vi "save_to_file.vi"(1 "Cell Settings Array 4":T1=[{"Measure?"=TRUE, "Area (cm^2)"=0.0, "Cell Label"="", "Cell Description"="", "Time between scans (s)"=0.0, "Cell Position"=1, "Scan settings in queue"=0, "Sample holder"=4.0, "User name"=""}, {"Measure?"=TRUE, "Area (cm^2)"=0.0, "Cell Label"="", "Cell Description"="", "Time between scans (s)"=0.0, "Cell Position"=2, "Scan settings in queue"=0, "Sample holder"=4.0, "User name"=""}, {"Measure?"=TRUE, "Area (cm^2)"=0.0, "Cell Label"="", "Cell Description"="", "Time between scans (s)"=0.0, "Cell Position"=3, "Scan settings in queue"=0, "Sample holder"=4.0, "User name"=""}, {"Measure?"=TRUE, "Area (cm^2)"=0.0, "Cell Label"="", "Cell Description"="", "Time between scans (s)"=0.0, "Cell Position"=4, "Scan settings in queue"=0, "Sample holder"=4.0, "User name"=""}, {"Measure?"=TRUE, "Area (cm^2)"=0.0, "Cell Label"="", "Cell Description"="", "Time between scans (s)"=0.0, "Cell Position"=5, "Scan settings in queue"=0, "Sample holder"=4.0, "User name"=""}, {"Measure?"=TRUE, "Area (cm^2)"=0.0, "Cell Label"="", "Cell Description"="", "Time between scans (s)"=0.0, "Cell Position"=6, "Scan settings in queue"=0, "Sample holder"=4.0, "User name"=""}, {"Measure?"=TRUE, "Area (cm^2)"=0.0, "Cell Label"="", "Cell Description"="", "Time between scans (s)"=0.0, "Cell Position"=7, "Scan settings in queue"=0, "Sample holder"=4.0, "User name"=""}, {"Measure?"=TRUE, "Area (cm^2)"=0.0, "Cell Label"="", "Cell Description"="", "Time between scans (s)"=0.0, "Cell Position"=8, "Scan settings in queue"=0, "Sample holder"=4.0, "User name"=""}, {"Measure?"=TRUE, "Area (cm^2)"=0.0, "Cell Label"="", "Cell Description"="", "Time between scans (s)"=0.0, "Cell Position"=9, "Scan settings in queue"=0, "Sample holder"=4.0, "User name"=""}, {"Measure?"=TRUE, "Area (cm^2)"=0.0, "Cell Label"="", "Cell Description"="", "Time between scans (s)"=0.0, "Cell Position"=10, "Scan settings in queue"=0, "Sample holder"=4.0, "User name"=""}, {"Measure?"=TRUE, "Area (cm^2)"=0.0, "Cell Label"="", "Cell Description"="", "Time between scans (s)"=0.0, "Cell Position"=11, "Scan settings in queue"=0, "Sample holder"=4.0, "User name"=""}, {"Measure?"=TRUE, "Area (cm^2)"=0.0, "Cell Label"="", "Cell Description"="", "Time between scans (s)"=0.0, "Cell Position"=12, "Scan settings in queue"=0, "Sample holder"=4.0, "User name"=""}, {"Measure?"=TRUE, "Area (cm^2)"=0.0, "Cell Label"="", "Cell Description"="", "Time between scans (s)"=0.0, "Cell Position"=13, "Scan settings in queue"=0, "Sample holder"=4.0, "User name"=""}, {"Measure?"=TRUE, "Area (cm^2)"=0.0, "Cell Label"="", "Cell Description"="", "Time between scans (s)"=0.0, "Cell Position"=14, "Scan settings in queue"=0, "Sample holder"=4.0, "User name"=""}, {"Measure?"=TRUE, "Area (cm^2)"=0.0, "Cell Label"="", "Cell Description"="", "Time between scans (s)"=0.0, "Cell Position"=15, "Scan settings in queue"=0, "Sample holder"=4.0, "User name"=""}, {"Measure?"=TRUE, "Area (cm^2)"=0.0, "Cell Label"="", "Cell Description"="", "Time between scans (s)"=0.0, "Cell Position"=16, "Scan settings in queue"=0, "Sample holder"=4.0, "User name"=""}] {"Scan settings in queue" items=["Standard"]}, 2 "Save Path":path) -> ()   [LabVIEW 2011]
uses:
  Typedefs/Cell details array.ctl
  Typedefs/Cell details cluster.ctl
  <vilib>/Utility/file.llb/Write To Spreadsheet File (string).vi
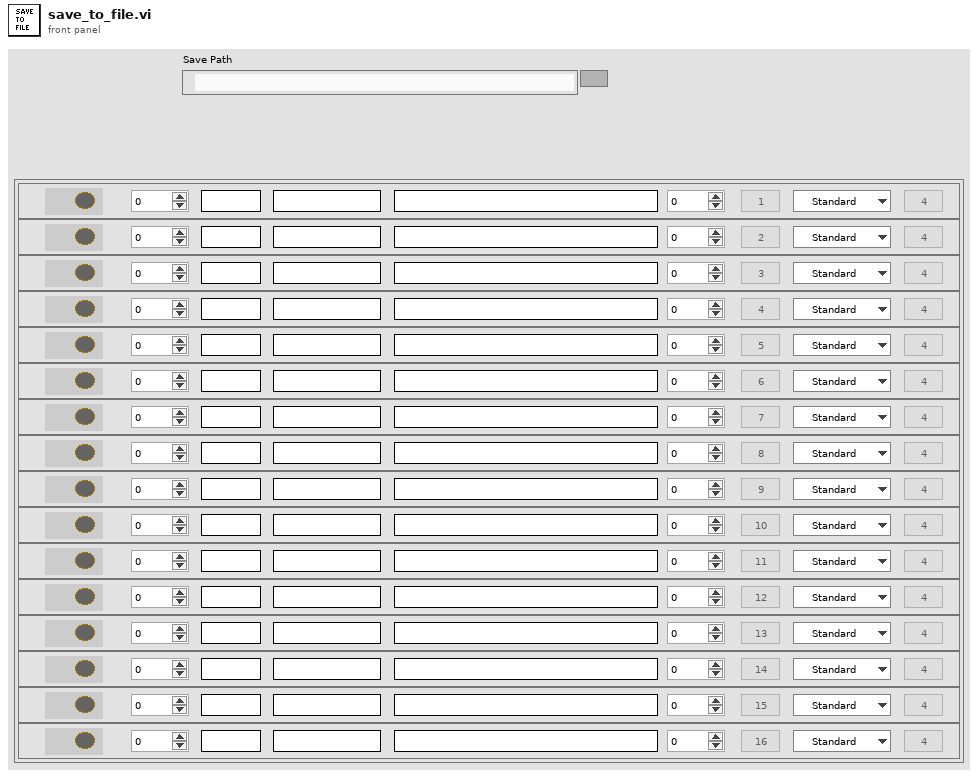
[diagram p1: front panel]
types:
  T1 = typedef "Cell details array.ctl" = T2[]
  T2 = typedef "Cell details cluster.ctl" = cluster{"Measure?":bool, "Area (cm^2)":dbl, "Cell Label":string, "Cell Description":string, "Time between scans (s)":dbl, "Cell Position":i32, "Scan settings in queue":u16, "Sample holder":dbl, "User name":string}
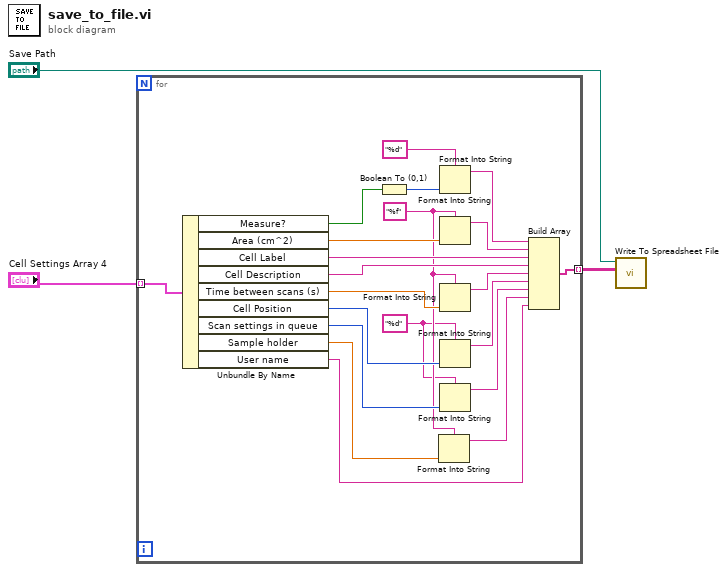
[diagram p0: block diagram]
diagram:
  n1 = for {
    tunnel: "Cell Settings Array 4" -> [w24] mode=indexing
    tunnel: [w11] -> w2 mode=indexing
    w6 = "%d" ("format string")
    w8 = "%f" ("format string")
    n2 = Unbundle By Name(w24) -> ("Measure?"=w23:bool, "Area (cm^2)"=w19:dbl, "Cell Label"=w17:string, "Cell Description"=w16:string, "Time between scans (s)"=w15:dbl, "Cell Position"=w13:i32, "Scan settings in queue"=w9:u16, "Sample holder"=w7:dbl, "User name"=w4:string)
    n3 = Boolean To (0,1)(Boolean=w23) -> (0, 1=w22:i16)
    n4 = Format Into String(format string=w8, w7) -> (resulting string=w5:string)  [unwired: 2 in, 1 out]
    n5 = Format Into String(format string="%d", w22) -> (resulting string=w20:string)  [unwired: 2 in, 1 out]
    n6 = Format Into String(format string=w8, w19) -> (resulting string=w18:string)  [unwired: 2 in, 1 out]
    n7 = Format Into String(format string=w8, w15) -> (resulting string=w14:string)  [unwired: 2 in, 1 out]
    n8 = Format Into String(format string=w6, w13) -> (resulting string=w12:string)  [unwired: 2 in, 1 out]
    n9 = Format Into String(format string=w6, w9) -> (resulting string=w10:string)  [unwired: 2 in, 1 out]
    n10 = Build Array(w20, w18, w17, w16, w14, w12, w10, w5, w4) -> (w11:string[])
  }
  n11 = call-poly <vilib>:"Write To Spreadsheet File.vi"("2D data"=w2, "file path (dialog if empty)"="Save Path") -> ()  [unwired: 6 in, 1 out]
